vi "SetAllPanesToOrigin.vi"(8 "error in":errorcluster, 10 "Panes":T1) -> (0 "error out":errorcluster)   [LabVIEW 2022 SP3, in "PentaPanesLibrary.lvlib" / "PentaPanes.lvclass"]
uses:
  PentaPanes.lvclass
  PanesCluster.ctl
  <vilib>/Utility/miscctls.llb/LVPointTypeDef.ctl
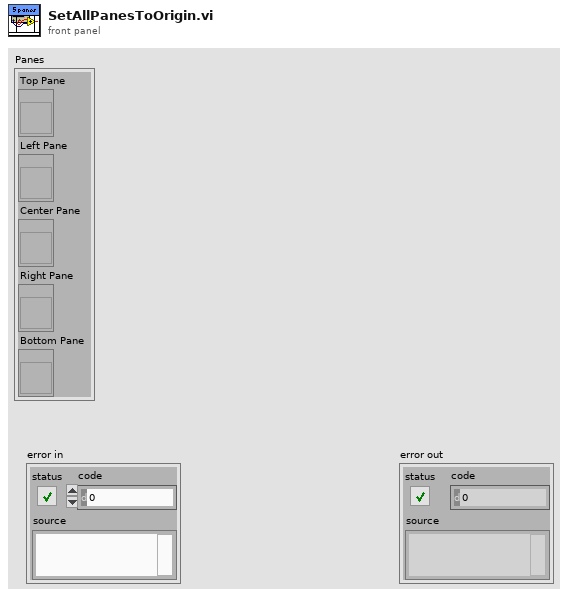
[diagram p1: front panel]
types:
  T1 = typedef "PentaPanesLibrary.lvlib/PentaPanes.lvclass/PanesCluster.ctl" = cluster{"Top Pane":refnum<vi>, "Left Pane":refnum<vi>, "Center Pane":refnum<vi>, "Right Pane":refnum<vi>, "Bottom Pane":refnum<vi>}
  T2 = typedef "LVPointTypeDef.ctl" = cluster{"Horizontal":i16, "Vertical":i16}
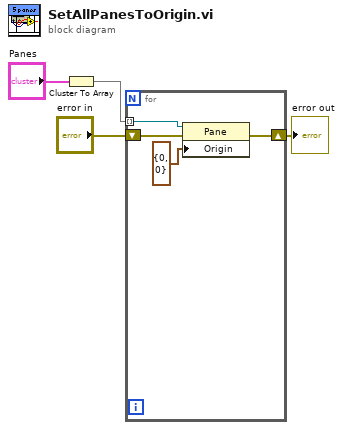
[diagram p0: block diagram]
diagram:
  n1 = Cluster To Array(cluster="Panes") -> (array=w2:refnum<vi>[])
  n2 = for {
    tunnel: w2 -> [w8] mode=indexing
    shift-right: [w6] -> w4
    shift-left: "error in" -> [w5]
    n3 = property class="Pane"(reference=w8, error in=w5, "Origin"=T2 {"Horizontal"=0, "Vertical"=0}) -> (error out=w6:errorcluster)  [unwired: 1 out]
  }
  "error out" <- w4
